vi "Test - Create from Ref Source.vi"() -> ()   [LabVIEW 2019]
doc: "This VI is used by the Create Control from Reference.vi example."
panel:
  in  "Source Cluster":T1
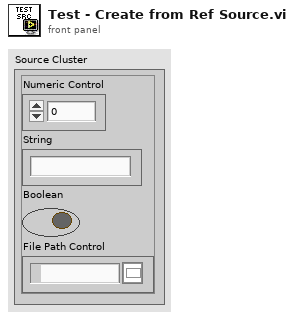
[diagram p1: front panel]
types:
  T1 = cluster{"Numeric Control":dbl, "String":string, "Boolean":bool, "File Path Control":path}
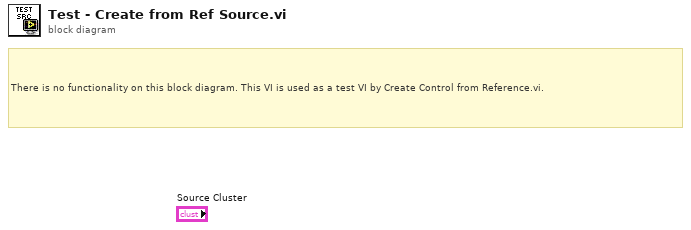
[diagram p0: block diagram]
diagram:
  # "There is no functionality on this block diagram. This VI is used as a test VI by Create Control from Reference.vi."
